vi "Configure_TW.vi"() -> (1 "changed?":bool, 2 "Property":string[](array[string]), 3 "Thing out":string)   [LabVIEW 2021]
uses:
  <vilib>/Utility/miscctls.llb/LVRowAndColumnUnsignedTypeDef.ctl
panel:
  in  "Delete  Property":bool
  in  "Add Property":bool
  in  "Login":bool
  in  "Properties":i32(listbox)
  in  "Cancel":bool
  in  "OK":bool
  in  "Thing":u16(ring) items=["Day1", "Day2"]
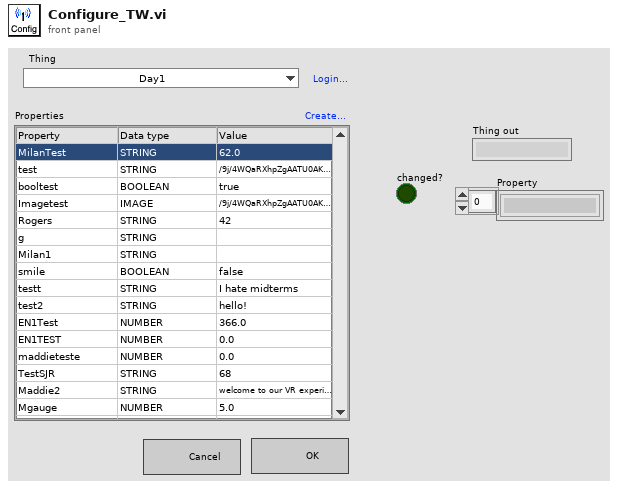
[diagram p1: front panel]
types:
  T1 = typedef "LVRowAndColumnUnsignedTypeDef.ctl" = cluster{"Row":u32, "Column":u32}
  T2 = enum16{"GET", "PUT", "POST", "MultiPOST", "DELETE"}
  T3 = cluster{"Name":string, "BaseURL":string, "AppKey":string, "Headers":string[], "Timeout":i32}
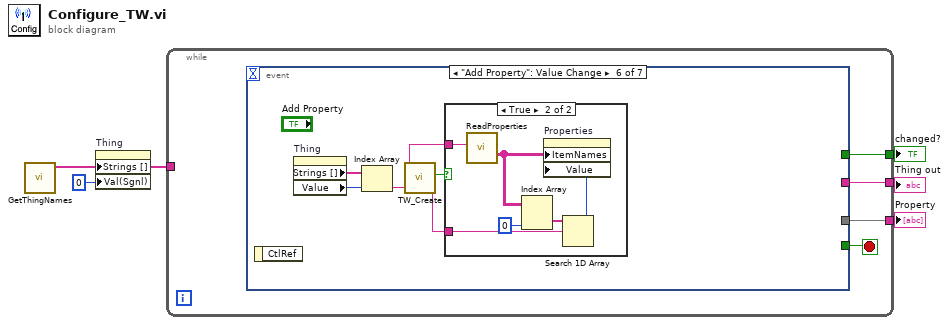
[diagram p0: block diagram]
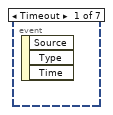
[diagram p2: hidden frame]
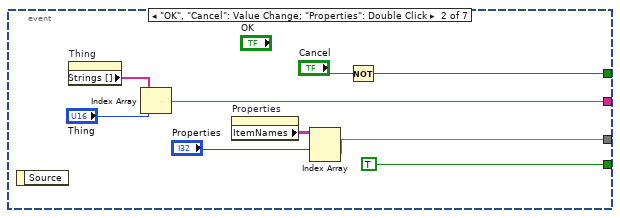
[diagram p3: hidden frame]
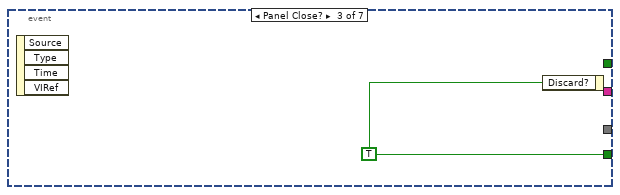
[diagram p4: hidden frame]
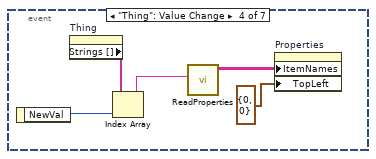
[diagram p5: hidden frame]
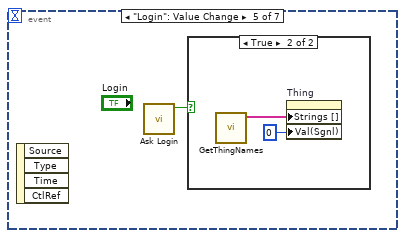
[diagram p6: hidden frame]
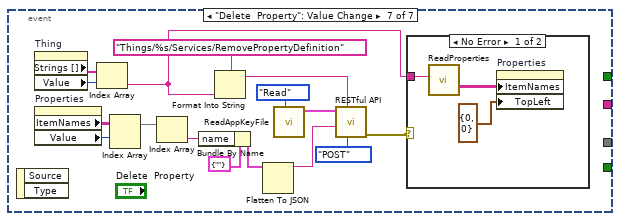
[diagram p9: hidden frame]
diagram:
  n1 = call "GetThingNames.vi"() -> ("Things"=w3:string[])  [unwired: 10 in, 1 out]
  n2 = property on="Thing" class="Ring (strict)"("Strings []"=w3, "Val(Sgnl)"=u16 0 ("Value (Signaling)")) -> ()  [unwired: 2 in, 2 out]
  n3 = while {
    tunnel: [w9] -> w4
    tunnel: w3 -> [_]
    tunnel: [w7] -> w2
    tunnel: [w6] -> w1
    stop <- w8 stop-if-true
    n4 = event shown="[5] \"Add Property\": Value Change" {
      selector: _ -> [_ _ _ _ _ _ _]
      dyn-events: _ -> [_ _ _ _ _ _ _]
      timeout: _ -> [_ _ _ _ _ _ _]
      tunnel: [_ w11 _ _ _ _ _] -> w9
      tunnel: [_ TRUE w19 _ _ _ _] -> w8
      tunnel: [_ w16 _ _ _ _ _] -> w7
      tunnel: [_ w13 _ _ _ _ _] -> w6
      event Timeout {
        n5 = event-data() -> ()  [unwired: 1 in, 3 out]
      }
      event "OK", "Cancel": Value Change; "Properties": Double Click {
        n6 = event-data() -> ()  [unwired: 1 in, 1 out]
        n7 = property on="Thing" class="Ring (strict)"() -> ("Strings []"=w10:string[])  [unwired: 2 in, 2 out]
        n8 = Index Array(array=w10, index="Thing") -> (element=w16:string)
        n9 = property on="Properties" class="MCListbox (strict)"() -> ("ItemNames"=w15:string[][])  [unwired: 2 in, 2 out]
        n10 = Index Array(array=w15, index (row)="Properties") -> (element=w13:string[])  [unwired: 1 in]
        n11 = Not(x="Cancel") -> (.not. x?=w11:bool)
      }
      event Panel Close? {
        w19 = TRUE
        n12 = event-data() -> ()  [unwired: 1 in, 4 out]
        n13 = event-data("Discard?"=w19) -> ()  [unwired: 1 in, 1 out]
      }
      event "Thing": Value Change {
        n14 = event-data() -> ("NewVal"=w24:u16)  [unwired: 1 in]
        n15 = property on="Thing" class="Ring (strict)"() -> ("Strings []"=w21:string[])  [unwired: 2 in, 2 out]
        n16 = Index Array(array=w21, index=w24) -> (element=w20:string)
        n17 = call "ReadProperties.vi"("Thing"=w20) -> ("All"=w23:string[][])  [unwired: 10 in]
        n18 = property on="Properties" class="MCListbox (strict)"("ItemNames"=w23, "TopLeft"=T1 {"Row"=0, "Column"=0} ("Top Left Visible Cell")) -> ()  [unwired: 2 in, 2 out]
      }
      event "Login": Value Change {
        n19 = event-data() -> ()  [unwired: 1 in, 4 out]
        n20 = call "Ask Login.vi"() -> ("OK?"=w25:bool)  [unwired: 10 in, 1 out]
        n21 = case shown="True" w25 {
          frame False {
          }
          frame True {
            n22 = call "GetThingNames.vi"() -> ("Things"=w27:string[])  [unwired: 10 in, 1 out]
            n23 = property on="Thing" class="Ring (strict)"("Strings []"=w27, "Val(Sgnl)"=u16 0 ("Value (Signaling)")) -> ()  [unwired: 2 in, 2 out]
          }
        }
      }
      event "Add Property": Value Change {
        n24 = event-data() -> ()  [unwired: 1 in, 1 out]
        n25 = property on="Thing" class="Ring (strict)"() -> ("Strings []"=w30:string[], "Value"=w31:u16)  [unwired: 2 in, 2 out]
        n26 = Index Array(array=w30, index=w31) -> (element=w29:string)
        n27 = call "TW_Create.vi"("Thingworx"=w29) -> ("Property out"=w28:string, "Success?"=w32:bool)  [unwired: 9 in]
        n28 = case shown="True" w32 {
          tunnel: w29 -> [_ w38]
          tunnel: w28 -> [_ w34]
          frame False {
          }
          frame True {
            n29 = call "ReadProperties.vi"("Thing"=w38) -> ("All"=w37:string[][])  [unwired: 10 in]
            n30 = Index Array(array=w37, index (col)=0 ("disabled index (col)")) -> (element=w35:string[])  [unwired: 1 in]
            n31 = Search 1D Array(1D array=w35, element=w34) -> (index of element=w33:i32)  [unwired: 1 in]
            n32 = property on="Properties" class="MCListbox (strict)"("ItemNames"=w37, "Value"=w33) -> ()  [unwired: 2 in, 2 out]
          }
        }
      }
      event "Delete  Property": Value Change {
        n33 = event-data() -> ()  [unwired: 1 in, 2 out]
        n34 = property on="Thing" class="Ring (strict)"() -> ("Strings []"=w48:string[], "Value"=w49:u16)  [unwired: 2 in, 2 out]
        n35 = property on="Properties" class="MCListbox (strict)"() -> ("ItemNames"=w46:string[][], "Value"=w47:i32)  [unwired: 2 in, 2 out]
        n36 = Index Array(array=w48, index=w49) -> (element=w43:string)
        n37 = Index Array(array=w46, index (row)=w47) -> (element=w45:string[])  [unwired: 1 in]
        n38 = Index Array(array=w45) -> (element=w40:string)  [unwired: 1 in]
        n39 = Bundle By Name(cluster=cluster{"name":string} {"name"=""}, "name"=w40) -> (w42:cluster{"name":string})
        n40 = Format Into String(format string="Things/%s/Services/RemovePropertyDefinition" ("url"), w43) -> (resulting string=w53:string)  [unwired: 2 in, 1 out]
        n41 = Flatten To JSON(anything=w42) -> (JSON string=w39:string)  [unwired: 2 in, 1 out]
        n42 = call "ReadAppKeyFile.vi"("Task"=enum16{"Read", "Write"}."Read") -> ("Device Out"=w54:T3)  [unwired: 8 in, 2 out]
        n43 = call "RESTful API.vi"("Method"=T2."POST", "url"=w53, "JSON"=w39, "Device In"=w54) -> ("error out"=w44:errorcluster)  [unwired: 5 in, 2 out]
        n44 = case shown="No Error" w44 {
          tunnel: w43 -> [w57 _]
          frame No Error {
            n45 = call "ReadProperties.vi"("Thing"=w57) -> ("All"=w55:string[][])  [unwired: 10 in]
            n46 = property on="Properties" class="MCListbox (strict)"("ItemNames"=w55, "TopLeft"=T1 {"Row"=0, "Column"=0} ("Top Left Visible Cell")) -> ()  [unwired: 2 in, 2 out]
          }
          frame Error {
          }
        }
      }
    }
  }
  "changed?" <- w4
  "Thing out" <- w2
  "Property" <- w1
